vi "#7.vi"(0 "System no.":i32=1 min=1 max=4 step=1, 5 "error in":errorcluster) -> (14 "Ready?":bool, 15 "String read":string, 19 "error out":errorcluster)   [LabVIEW 2020]
doc: "Sends the single ASCII character 7 and returns the ready status of the controller. Sub-VI for Wait for answer of longlasting command.vi.\n\nC-880K005: VI only supported when called through PI_Multix.vi\n\nC-887, F-206, M-8X0: Only for GCS syntax version = GCS 2.0 or higher (check with CSV?.vi. If CSV?.vi is not supported, syntax version is GCS 1.0).\n\nE-712: This VI is to be used during reference moves only."
panel:
  # "Sends ASCII #7 without LineFeed and returns the ready status of the controller."
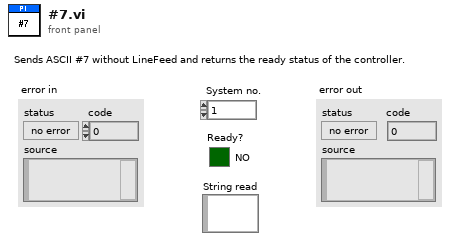
[diagram p1: front panel]
types:
  T1 = enum16{"Disable error check", "Force error check", "Use global settings"}
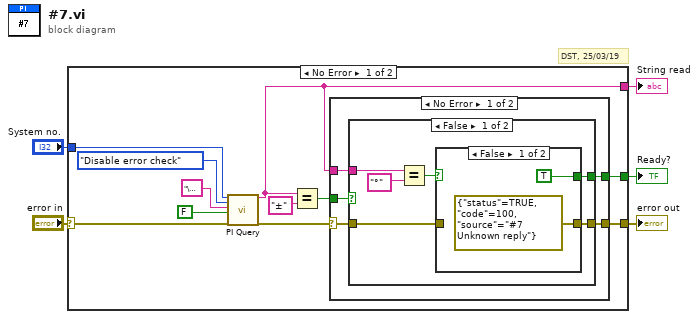
[diagram p0: block diagram]
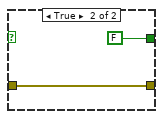
[diagram p2: hidden frame]
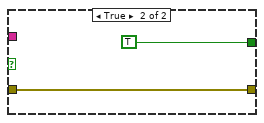
[diagram p3: hidden frame]
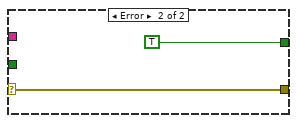
[diagram p4: hidden frame]
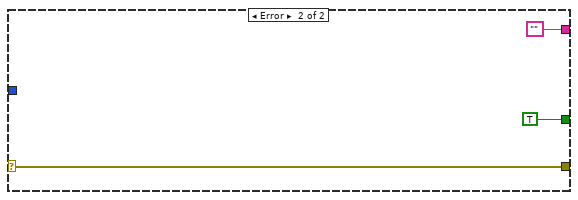
[diagram p5: hidden frame]
diagram:
  # "DST, 25/03/19"
  n1 = case shown="No Error" "error in" {
    selector: "error in" -> [w7 w38]
    tunnel: "System no." -> [w14 _]
    tunnel: [w12 w38] -> w4
    tunnel: [w11 TRUE] -> w3
    tunnel: [w9 ""] -> w2
    frame No Error {
      n2 = call "PI Query.vi"("System no."=w14, "Error check settings"=T1."Disable error check", "String to send"="\u0007", "Attach termination char.?"=FALSE ("Attach Linefeed?"), "error in"=w7) -> ("String read"=w9:string, "error out"=w8:errorcluster)  [unwired: 2 in, 11 out]
      n3 = Equal?(x=w9, y="±" ("String read")) -> (x = y?=w13:bool)
      n4 = case shown="No Error" w8 {
        selector: w8 -> [w17 w34]
        tunnel: w13 -> [w21 _]
        tunnel: [w20 w34] -> w12
        tunnel: [w19 TRUE] -> w11
        tunnel: w9 -> [w18 _]
        frame No Error {
          n5 = case shown="False" w21 {
            tunnel: w17 -> [w24 w33]
            tunnel: [w23 w33] -> w20
            tunnel: [w25 TRUE] -> w19
            tunnel: w18 -> [w27 _]
            frame False {
              n6 = Equal?(x=w27, y="°" ("String read")) -> (x = y?=w26:bool)
              n7 = case shown="False" w26 {
                tunnel: [TRUE FALSE] -> w25
                tunnel: w24 -> [_ w30]
                tunnel: [errorcluster {"status"=TRUE, "code"=100, "source"="#7 Unknown reply"} ("error out") w30] -> w23
                frame False {
                }
                frame True {
                }
              }
            }
            frame True {
            }
          }
        }
        frame Error {
        }
      }
    }
    frame Error {
    }
  }
  "error out" <- w4
  "Ready?" <- w3
  "String read" <- w2
